vi "Read True by Reference.vi"(8 "Error In":errorcluster, 11 "Reader In":refnum<data-value>) -> (0 "Error Out":errorcluster, 3 "Reader Out":refnum<data-value>)   [LabVIEW 2018, in "Toolkit.lvlib" / "Reader.lvclass"]
uses:
  Reader.lvclass
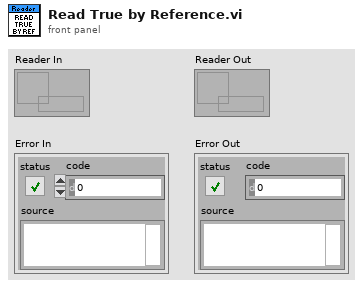
[diagram p1: front panel]
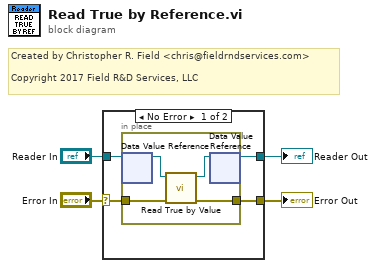
[diagram p0: block diagram]
diagram:
  # "Created by Christopher R. Field <chris@fieldrndservices.com>\n\nCopyright 2017 Field R&D Services, LLC"
  n1 = case shown="No Error" "Error In" {
    selector: "Error In" -> [w6 w13]
    tunnel: "Reader In" -> [w8 w14]
    tunnel: [w7 w14] -> w3
    tunnel: [w5 w13] -> w1
    frame No Error {
      n2 = in-place {
        in-place-border: w6 -> [w10]
        in-place-border: [w9] -> w5
        n3 = in-place-dvr #1(w8) -> (w12:refnum<class "Reader.lvclass">)  [unwired: 1 out]
        n4 = call "Read True by Value.vi"("Error In"=w10, "Reader In"=w12) -> ("Error Out"=w9:errorcluster, "Reader Out"=w11:refnum<class "Reader.lvclass">)  [unwired: 8 in]
        n5 = in-place-dvr #1(w11) -> (w7:refnum<data-value>)  [unwired: 1 out]
      }
    }
    frame Error {
    }
  }
  "Reader Out" <- w3
  "Error Out" <- w1
